vi "Registry Actions Event.vi"() -> ()   [LabVIEW 2018, in "GLog.lvlib" / "Registry.lvlib"]
uses:
  Registry.lvlib
  Registry Message.ctl
  Registry Actions.ctl
panel:
  in  "registry vi":refnum<vi>
  in  "registry actions":refnum<user-event>
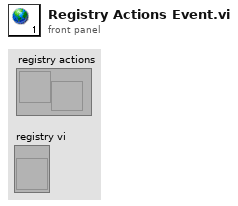
[diagram p1: front panel]
diagram:
